vi "MISC Create Start_End Time.vi"(11 "Error In (no error)":errorcluster) -> (4 "Time":string, 15 "Error Out":errorcluster)   [LabVIEW 2011]
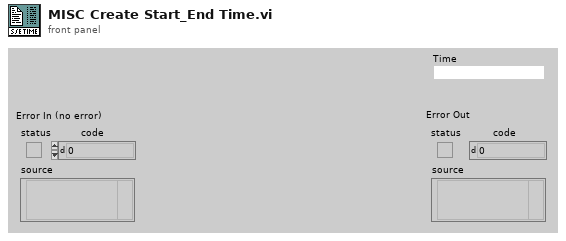
[diagram p1: front panel]
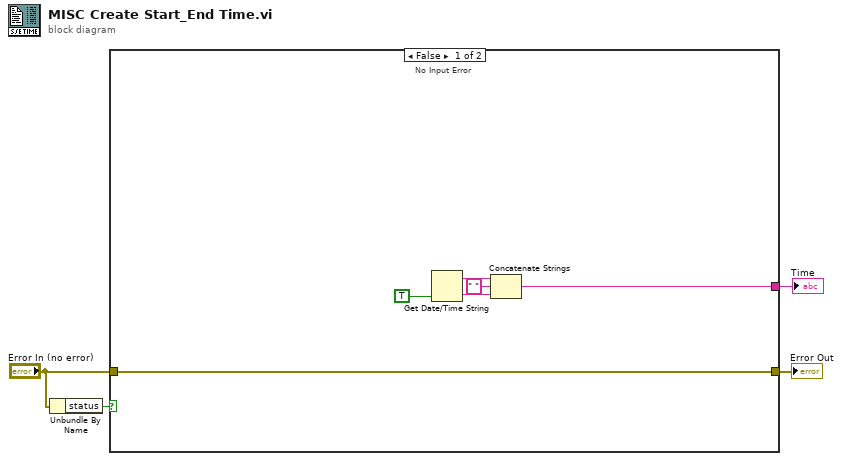
[diagram p0: block diagram]
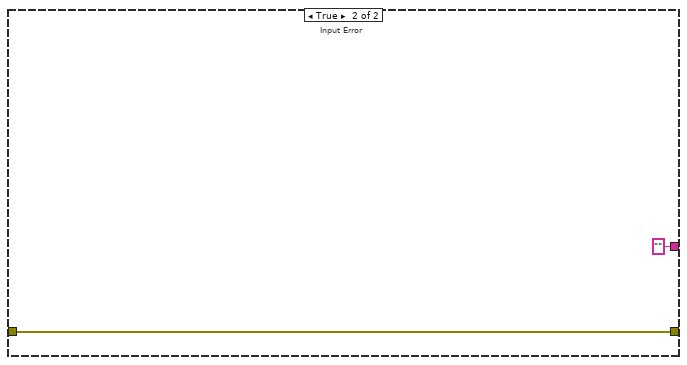
[diagram p2: hidden frame]
diagram:
  n1 = Unbundle By Name("Error In (no error)") -> ("status"=w4:bool)
  n2 = case shown="False" w4 {
    tunnel: [w10 w12] -> w3
    tunnel: "Error In (no error)" -> [w10 w12]
    tunnel: [w5 ""] -> w1
    frame False {
      # "No Input Error"
      n3 = Get Date/Time String(want seconds? (F)=TRUE) -> (date string=w9:string, time string=w8:string)  [unwired: 2 in]
      n4 = Concatenate Strings(w9, " " ("Substring"), w8) -> (w5:string)
    }
    frame True {
      # "Input Error"
    }
  }
  "Error Out" <- w3
  "Time" <- w1
